vi "calibrateRFAmp.vi"(8 "error in (no error)":errorcluster, 9 "amplitude":string, 10 "channel_name":string, 11 "ChannelArray in":refnum<class "ChannelArray.lvclass">) -> (0 "error out":errorcluster, 2 "amplitude":dbl, 3 "ChannelArray out":refnum<class "ChannelArray.lvclass">)   [LabVIEW 2011, in "Tools.lvlib" / "DatabaseHelpers.lvlib" / "ChannelArray.lvclass"]
uses:
  ChannelArray.lvclass
  Channel/RfOutputChannel/RfOutputChannel.lvclass
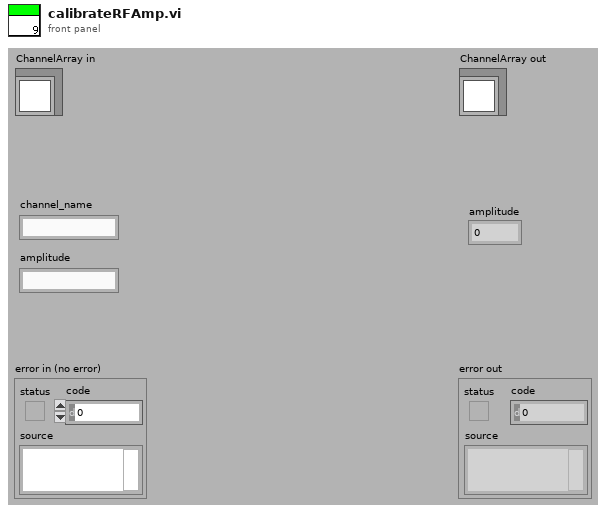
[diagram p1: front panel]
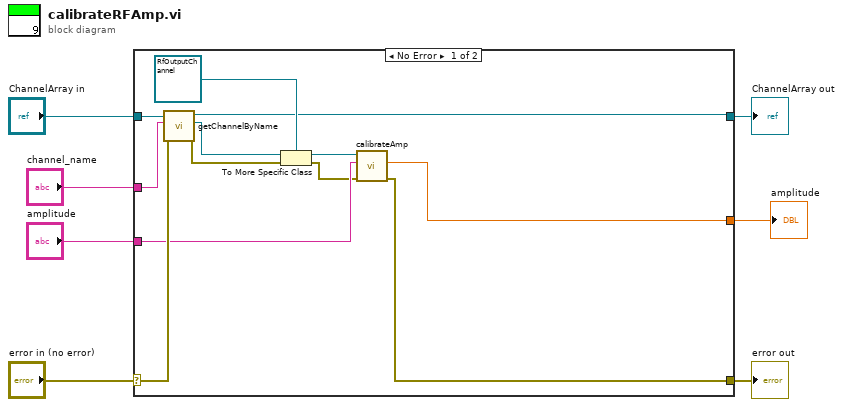
[diagram p0: block diagram]
diagram:
  n1 = case shown="No Error" "error in (no error)" {
    selector: "error in (no error)" -> [w17 w21]
    tunnel: [w8 w21] -> w6
    tunnel: [w10 w20] -> w4
    tunnel: "ChannelArray in" -> [w19 w20]
    tunnel: "channel_name" -> [w18 _]
    tunnel: "amplitude" -> [w13 _]
    tunnel: [w9 _] -> w1
    frame No Error {
      n2 = call-dynamic "getChannelByName.vi"("error in (no error)"=w17, "channel_name"=w18, "ChannelArray in"=w19) -> ("error out"=w11:errorcluster, "Channel"=w15:refnum<class "Channel.lvclass">, "ChannelArray out"=w10:refnum<class "ChannelArray.lvclass">)  [unwired: 5 in, 1 out]
      n3 = To More Specific Class(target class=refnum<class "RfOutputChannel.lvclass"> refnum ("RfOutputChannel in"), reference=w15, error in=w11) -> (specific class reference=w14:refnum<class "RfOutputChannel.lvclass">, error out=w12:errorcluster)
      n4 = call "calibrateAmp.vi"("error in (no error)"=w12, "value"=w13, "RfOutputChannel in"=w14) -> ("error out"=w8:errorcluster, "Amplitude"=w9:dbl)  [unwired: 6 in, 1 out]
    }
    frame Error {
    }
  }
  "error out" <- w6
  "ChannelArray out" <- w4
  "amplitude" <- w1
